vi "Update Bored Operation.vi"(0 "Monkeys in":T1, 1 "Bored Operation":string) -> (2 "Monkeys out":T1)   [LabVIEW 2020, in "AoC 2022.lvlib"]
uses:
  AoC 2022.lvlib
  Monkey.ctl
  Monkeys.ctl
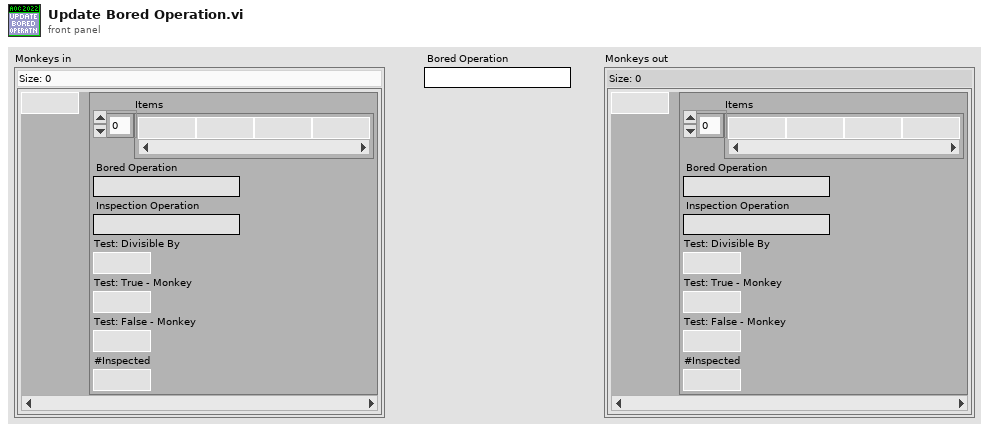
[diagram p1: front panel]
types:
  T1 = typedef "AoC 2022.lvlib/Monkeys.ctl" = map{i32, T2}
  T2 = typedef "AoC 2022.lvlib/Monkey.ctl" = cluster{"Items":u64[], "Bored Operation":string, "Inspection Operation":string, "Test: Divisible By":u64, "Test: True - Monkey":i32, "Test: False - Monkey":i32, "#Inspected":i32}
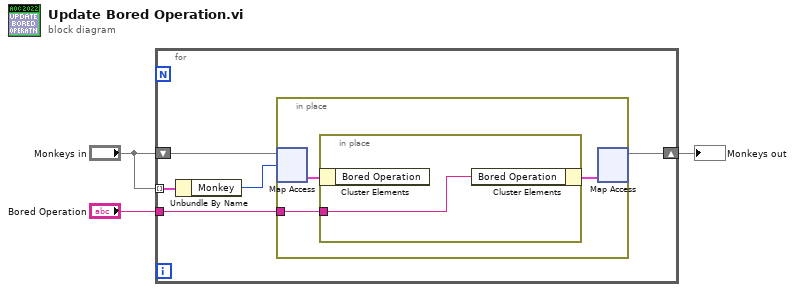
[diagram p0: block diagram]
diagram:
  n1 = for {
    shift-right: [w5] -> w2
    shift-left: "Monkeys in" -> [w8]
    tunnel: "Monkeys in" -> [w7] mode=indexing
    tunnel: "Bored Operation" -> [w4]
    n2 = Unbundle By Name(w7) -> ("Monkey"=w6:i32)
    n3 = in-place {
      in-place-border: w4 -> [w9]
      n4 = in-place-map #1(w8, w6) -> (w11:T2)  [unwired: 1 in, 1 out]
      n5 = in-place {
        in-place-border: w9 -> [w12]
        n6 = in-place-cluster #2(w11) -> ()  [unwired: 1 out]
        n7 = in-place-cluster #2("Bored Operation"=w12) -> (w10:T2)
      }
      n8 = in-place-map #1(w10) -> (w5:T1)  [unwired: 1 in, 2 out]
    }
  }
  "Monkeys out" <- w2
